vi "shag_start — 5.vi"() -> ()   [LabVIEW 2016]
uses:
  <vilib>/Instr/_visa.llb/VISA Configure Serial Port (Instr).vi
panel:
  out "file":i32
  out "положение в мин 1":i32
  in  "stop":bool
  in  "all":T1(tab)
  out "положение шд":i32(knob) scale=-10.0..190.0
  out "текущее положение":string
  out "положение в минутах 1":string
  in  "Минуты":i32 min=-600 max=11400
  in  "Stop двигатель":bool
  in  "Вращение по градусам +":bool
  in  "Вращение по градусам -":bool
  in  "Вернуться в нулевое положение":bool
  in  "Задать текущее положение нулевым":bool
  in  "Установка минут":bool
  in  "Блокировать зеркало №1":bool
  in  "Выберете COM порт":refnum<visa-resource-name>="COM1"
  in  "Скорость обмена данными":u32(ring)=19200 items=["9600"=9600, "19200"=19200, "38400"=38400, "57600"=57600]
  in  "Число бит на символ":u16=8 min=5 max=8 step=1
  in  "Контроль чётности":enum16{"None", "Odd", "Even", "Mark", "Space"}(ring)
  in  "Стоповый бит":u16(ring)=10 items=["1.0"=10, "1.5"=15, "2.0"=20]
  in  "Контроль переполнения":u16(ring) items=["None"=0, "XON/XOFF"=1, "RTS/CTS"=2, "DTR/DSR"=4]
  # "1 - адресс 1 двигателя\n2 - адресс 2 двигателя\n$0MV\\01+   - запуск всех двигателей в положительном направлении \n$0MS\\00   - остановка всех двигателей\n$0MJ\\04+\\00\\00\\01   - 1 шаг всех двигателей\n$0SS\\01\\10   - скорость 10 для всех двигателей"
  # "Зеркало №1:"
  # "Положение:"
  # "Ренгеновская трубка №2:"
  # "Положение ренгеновской трубк:"
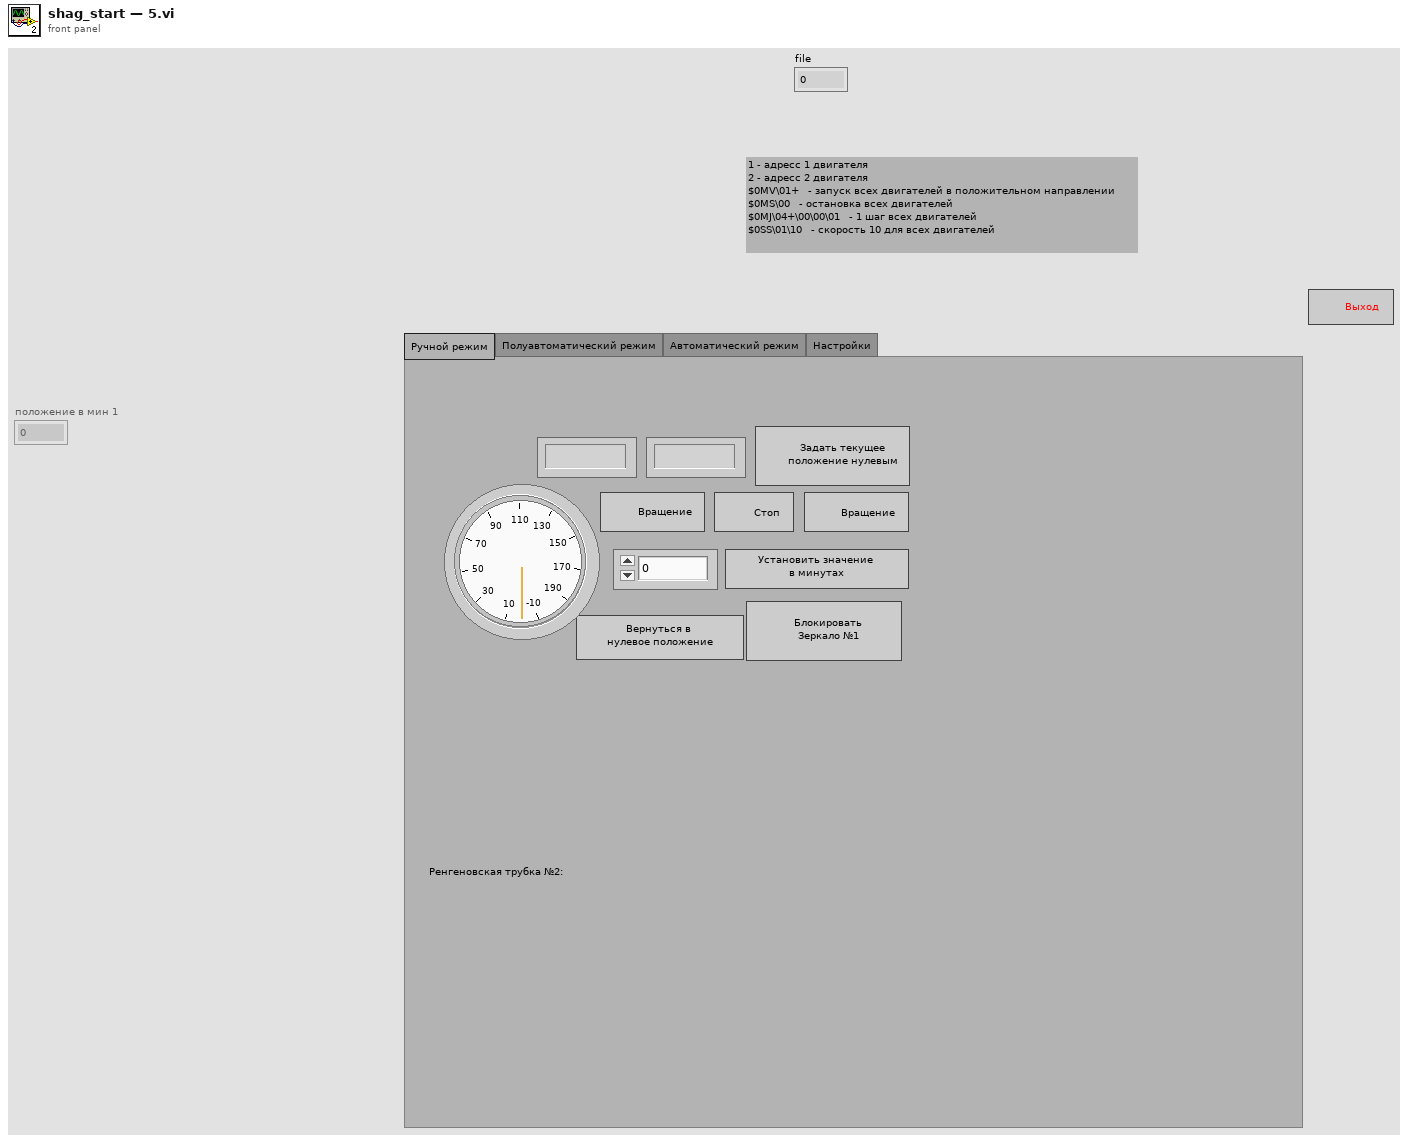
[diagram p1: front panel]
types:
  T1 = enum32{"Ручной режим", "Полуавтоматический режим", "Автоматический режим", "Настройки"}
  T2 = enum16{"open", "replace", "create", "open or create", "replace or create", "replace or create with confirmation"}
  T3 = enum8{"Enabled", "Disabled", "Disabled and Grayed Out"}
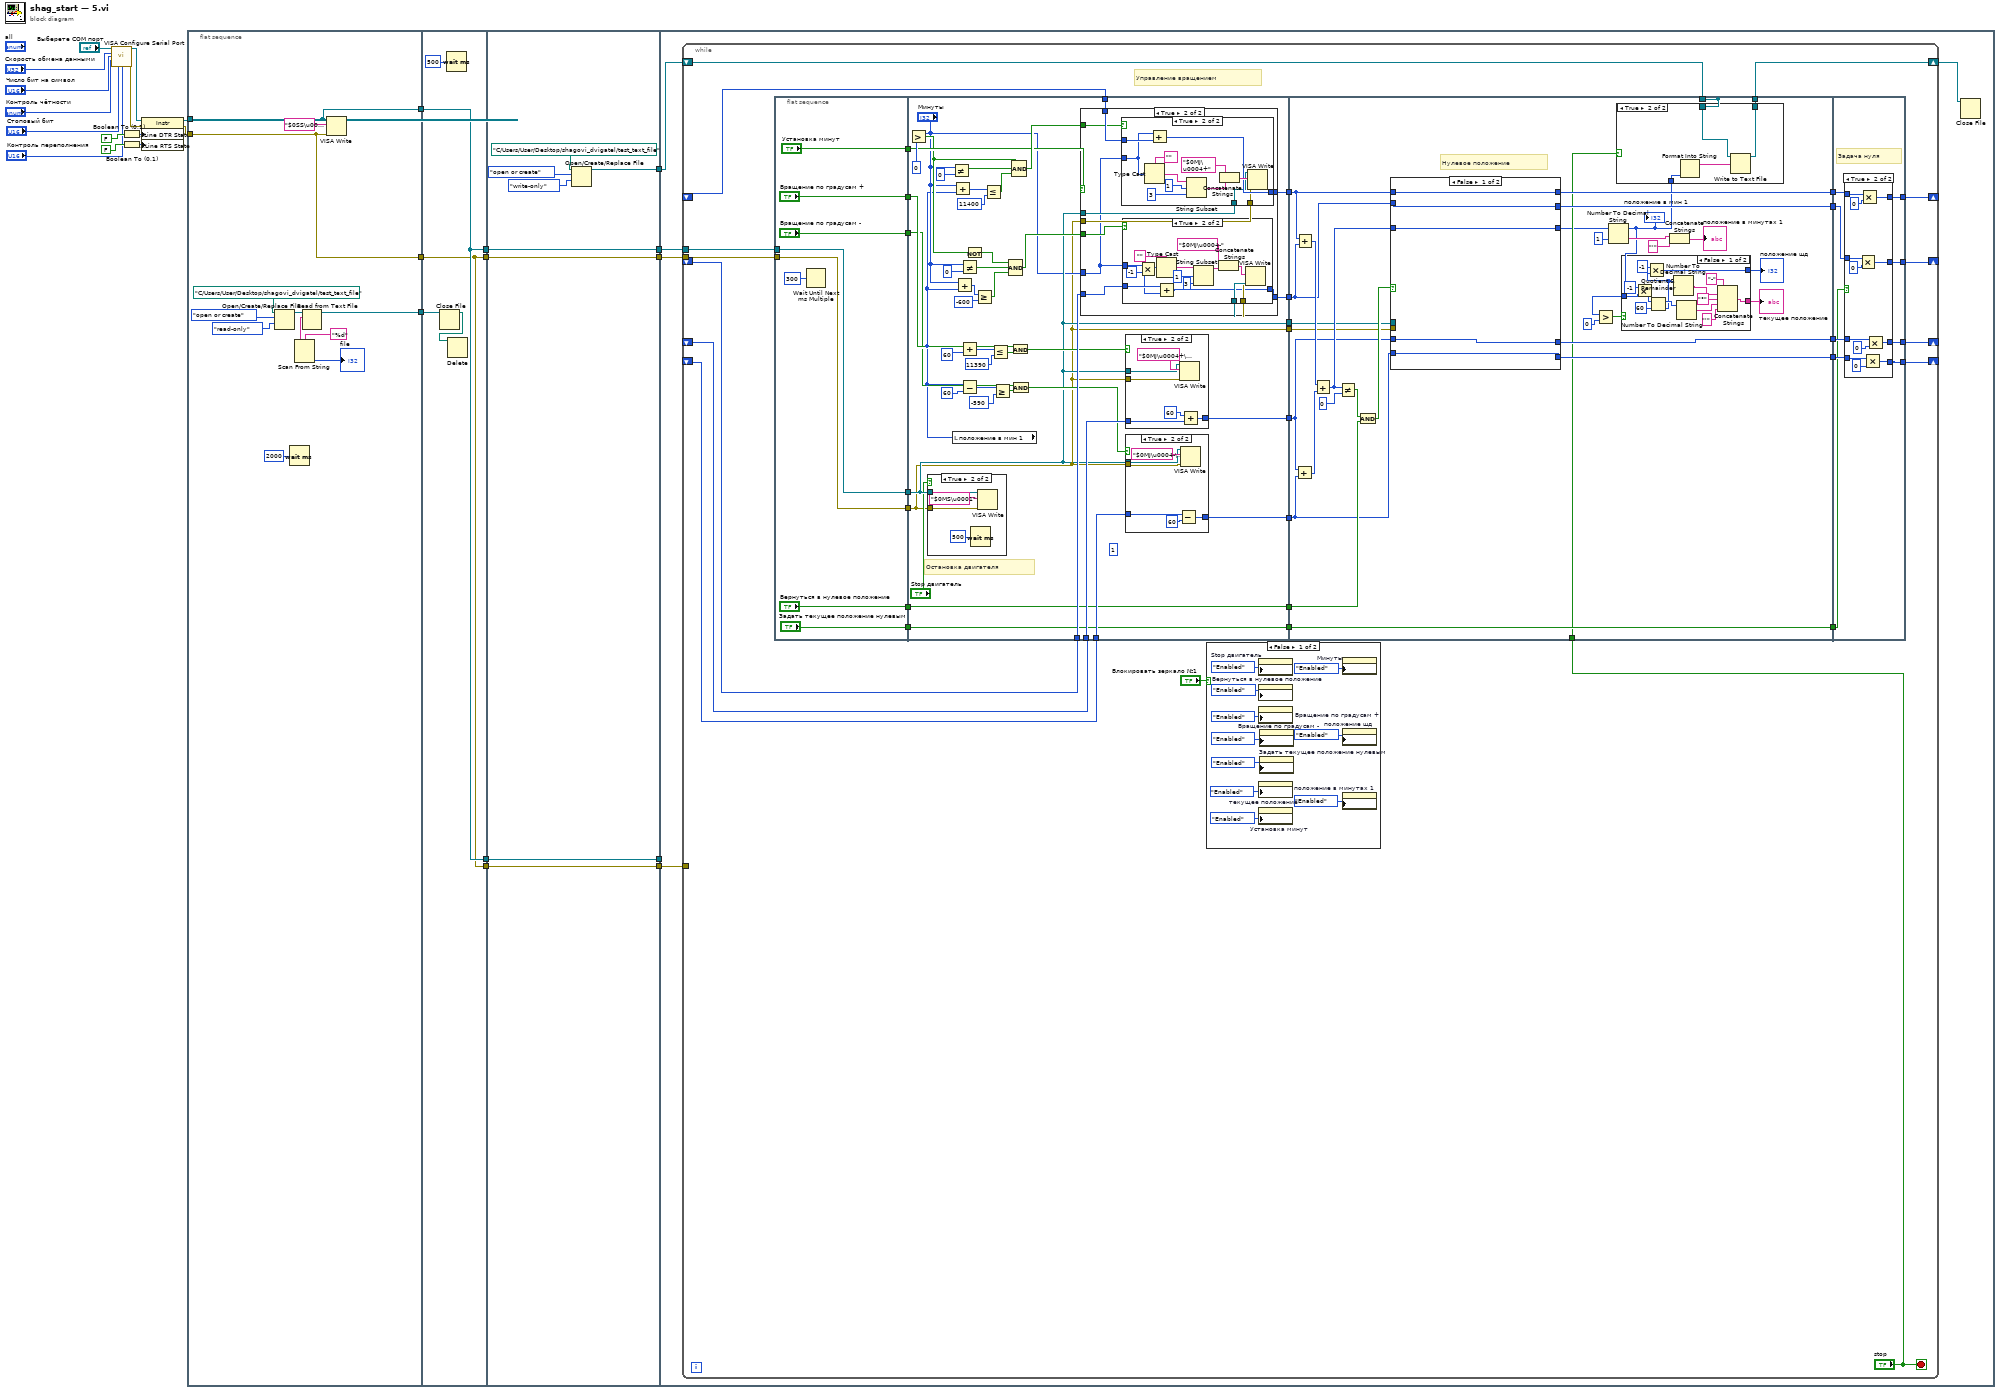
[diagram p0: block diagram]
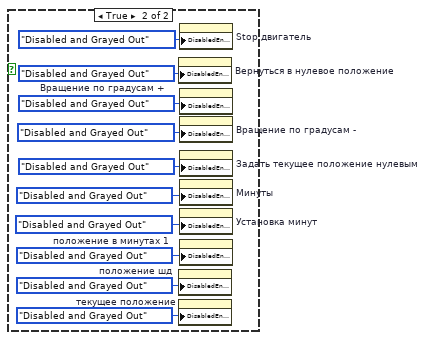
[diagram p2: hidden frame]
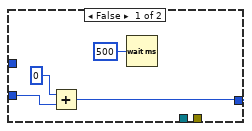
[diagram p4: hidden frame]
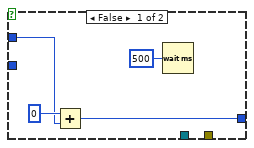
[diagram p5: hidden frame]
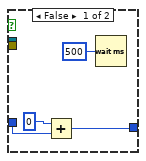
[diagram p7: hidden frame]
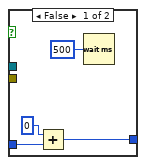
[diagram p8: hidden frame]
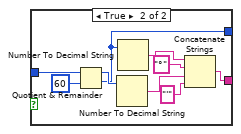
[diagram p10: hidden frame]
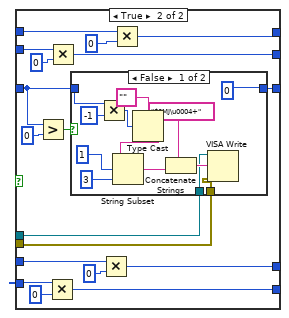
[diagram p11: hidden frame]
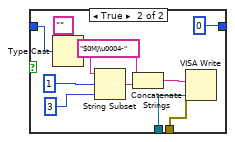
[diagram p12: hidden frame]
diagram:
  n1 = call-poly "VISA Configure Serial Port"("VISA resource name"="Выберете COM порт", "baud rate (9600)"="Скорость обмена данными", "data bits (8)"="Число бит на символ", "parity (0:none)"="Контроль чётности", "stop bits (10: 1 bit)"="Стоповый бит", "flow control (0:none)"="Контроль переполнения") -> ("VISA resource name out"=w24:refnum<visa-resource-name>, "error out"=w23:errorcluster)  [unwired: 8 in]
  n2 = Boolean To (0,1)(Boolean=FALSE ("DTR Write")) -> (0, 1=w25:i16)
  n3 = Boolean To (0,1)(Boolean=FALSE ("DTR Write")) -> (0, 1=w26:i16)
  n4 = property class="Instr"(reference=w24, error in=w23, "Serial Settings:Modem Line Settings:Line DTR State"=w25, "Serial Settings:Modem Line Settings:Line RTS State"=w26) -> (reference out=w22:refnum<visa-resource-name>, error out=w21:errorcluster)
  n5 = flat-sequence {
    tunnel: w22 -> [w37]
    tunnel: w21 -> [w36]
    tunnel: [w37] -> w20
    tunnel: [w36] -> w19
    tunnel: [w30] -> w10
    tunnel: [w42] -> w9
    tunnel: w20 -> [w42]
    tunnel: w19 -> [w41]
    tunnel: [w41] -> w7
    tunnel: [w42] -> w5
    tunnel: [w41] -> w3
    tunnel: w10 -> [w40]
    tunnel: w9 -> [w51]
    tunnel: [w51] -> w8
    tunnel: w7 -> [w50]
    tunnel: [w50] -> w6
    tunnel: w5 -> [w49]
    tunnel: [w49] -> w4
    tunnel: w3 -> [w48]
    tunnel: [w48] -> w2
    tunnel: [w44] -> w1
    tunnel: w8 -> [w56]
    tunnel: w6 -> [w55]
    tunnel: w4 -> [_]
    tunnel: w2 -> [w54]
    tunnel: w1 -> [w53]
    frame #0 {
      n6 = Open/Create/Replace File(file path (use dialog)=path "C:/Users/User/Desktop/shagovi_dvigatel/test_text_file", operation (0:open)=T2."open or create", access (0:read/write)=enum16{"read/write", "read-only", "write-only"}."read-only") -> (refnum out=w29:refnum<file>)  [unwired: 3 in, 2 out]
      n7 = Wait (ms)(milliseconds to wait=u32 2000) -> ()  [unwired: 1 out]
      n8 = Read from Text File(file (use dialog)=w29) -> (refnum out=w30:refnum<file>, text=w33:string)  [unwired: 3 in, 2 out]
      n9 = Scan From String(format string="%d", input string=w33) -> (output 1=→"file":i32)  [unwired: 3 in, 3 out]
      n10 = VISA Write(VISA resource name=w37, write buffer="$0SS\u0001\u0010", error in (no error)=w36) -> ()  [unwired: 3 out]
    }
    frame #1 {
      n11 = Close File(refnum=w40) -> (path=w39:path)  [unwired: 1 in, 1 out]
      n12 = Wait (ms)(milliseconds to wait=u32 500) -> ()  [unwired: 1 out]
      n13 = Delete(path (use dialog)=w39) -> ()  [unwired: 4 in, 3 out]
    }
    frame #2 {
      n14 = Open/Create/Replace File(file path (use dialog)=path "C:/Users/User/Desktop/shagovi_dvigatel/test_text_file", operation (0:open)=T2."open or create", access (0:read/write)=enum16{"read/write", "read-only", "write-only"}."write-only") -> (refnum out=w44:refnum<file>)  [unwired: 3 in, 2 out]
    }
    frame #3 {
      n15 = while {
        tunnel: w56 -> [w66]
        tunnel: w55 -> [w65]
        shift-right: [w61] -> _
        shift-left: _ -> [w70]
        shift-right: [w62] -> _
        shift-left: _ -> [w69]
        shift-right: [w63] -> _
        shift-left: _ -> [w68]
        shift-right: [w64] -> _
        shift-left: _ -> [w67]
        tunnel: w54 -> [_]
        shift-right: [w57] -> w52
        shift-left: w53 -> [w58]
        stop <- "stop" stop-if-true
        # "Управление вращением"
        n16 = flat-sequence {
          tunnel: w65 -> [w117]
          tunnel: w66 -> [w118]
          tunnel: [w118] -> w90
          tunnel: [w117] -> w89
          tunnel: ["Вращение по градусам +"] -> w88
          tunnel: ["Вращение по градусам -"] -> w87
          tunnel: ["Вернуться в нулевое положение"] -> w86
          tunnel: ["Задать текущее положение нулевым"] -> w85
          tunnel: ["Установка минут"] -> w84
          tunnel: w90 -> [w138]
          tunnel: w89 -> [w120]
          tunnel: [w161] -> w83
          tunnel: w70 -> [w158]
          tunnel: w69 -> [w160]
          tunnel: [w159] -> w82
          tunnel: w68 -> [w157]
          tunnel: w67 -> [w156]
          tunnel: w88 -> [w142]
          tunnel: w87 -> [w141]
          tunnel: [w155] -> w81
          tunnel: [w154] -> w80
          tunnel: [w139] -> w79
          tunnel: w86 -> [w139]
          tunnel: [w120] -> w78
          tunnel: [w138] -> w77
          tunnel: [w137] -> w76
          tunnel: w85 -> [w137]
          tunnel: w84 -> [w131]
          tunnel: w83 -> [w239]
          tunnel: w82 -> [w240]
          tunnel: [w260] -> w75
          tunnel: [w258] -> w74
          tunnel: w81 -> [w241]
          tunnel: w80 -> [w242]
          tunnel: [w248] -> w73
          tunnel: [w256] -> w72
          tunnel: w79 -> [w252]
          tunnel: w78 -> [w247]
          tunnel: w77 -> [w246]
          tunnel: w76 -> [w244]
          tunnel: [w244] -> w71
          tunnel: [w233] -> _
          tunnel: "stop" -> [w236]
          tunnel: w58 -> [w233]
          tunnel: [w232] -> w57
          tunnel: [w344] -> w61
          tunnel: [w341] -> w62
          tunnel: w75 -> [w343]
          tunnel: w74 -> [w342]
          tunnel: [w340] -> w63
          tunnel: [w339] -> w64
          tunnel: w73 -> [w338]
          tunnel: w72 -> [w337]
          tunnel: w71 -> [w336]
          frame #0 {
            n17 = Wait Until Next ms Multiple(millisecond multiple=u32 300) -> ()  [unwired: 1 out]
          }
          frame #1 {
            (unwired) 1
            # "Остановка двигателя"
            n18 = Greater?(x="Минуты", y=0) -> (0:w129:bool)
            n19 = case shown="True" "Stop двигатель" {
              tunnel: w138 -> [_ w208]
              tunnel: w120 -> [_ w207]
              frame False {
              }
              frame True {
                n20 = Wait (ms)(milliseconds to wait=u32 500) -> ()  [unwired: 1 out]
                n21 = VISA Write(VISA resource name=w208, write buffer="$0MS\u0001", error in (no error)=w207) -> ()  [unwired: 3 out]
              }
            }
            n22 = Not Equal?(x="Минуты", y=0) -> (x != y?=w128:bool)
            n23 = local read "положение в мин 1"() -> (w119:i32)
            n24 = Add(x="Минуты", y=w119) -> (x+y=w152:i32)
            n25 = Add(x="Минуты", y=w119) -> (x+y=w123:i32)
            n26 = Not Equal?(x="Минуты", y=0) -> (x != y?=w126:bool)
            n27 = Add(x=w119, y=60) -> (x+y=w147:i32)
            n28 = Subtract(x=w119, y=60) -> (x-y=w134:i32)
            n29 = Not(x=w129) -> (.not. x?=w130:bool)
            n30 = Greater Or Equal?(x=w123, y=-600) -> (x >= y?=w124:bool)
            n31 = Less Or Equal?(x=w152, y=11400) -> (x <= y?=w127:bool)
            n32 = Less Or Equal?(x=w147, y=11390) -> (x <= y?=w144:bool)
            n33 = Greater Or Equal?(x=w134, y=-590) -> (x >= y?=w135:bool)
            n34 = Compound Arithmetic op=AND(w130, w126, w124) -> (w148:bool)
            n35 = And(x=w142, y=w144) -> (x .and. y?=w143:bool)
            n36 = And(x=w141, y=w135) -> (x .and. y?=w140:bool)
            n37 = Compound Arithmetic op=AND(w129, w128, w127) -> (w150:bool)
            n38 = case shown="True" w131 {
              tunnel: [w163 w172] -> w161
              tunnel: w160 -> [w162 w171]
              tunnel: [w162 w170] -> w159
              tunnel: w158 -> [w163 w169]
              tunnel: w150 -> [_ w168]
              tunnel: w148 -> [_ w167]
              tunnel: w120 -> [_ w166]
              tunnel: w138 -> [_ w165]
              tunnel: "Минуты" -> [_ w164]
              frame False {
              }
              frame True {
                n39 = case shown="True" w168 {
                  tunnel: [w193 w199] -> w172
                  tunnel: w169 -> [w192 w198]
                  tunnel: w166 -> [_ w197]
                  tunnel: w165 -> [_ w196]
                  tunnel: w164 -> [_ w195]
                  frame False {
                    n40 = Add(x=0, y=w192) -> (x+y=w193:i32)
                    n41 = Wait (ms)(milliseconds to wait=u32 500) -> ()  [unwired: 1 out]
                  }
                  frame True {
                    n42 = Type Cast(type="", x=w195) -> (*(type *) &x=w202:string)
                    n43 = Add(x=w195, y=w198) -> (x+y=w199:i32)
                    n44 = String Subset(string=w202, offset (0)=1, length (rest)=3 ("length (rest)")) -> (substring=w201:string)
                    n45 = Concatenate Strings("$0MJ\u0004+" ("write buffer"), w201) -> (w205:string)
                    n46 = VISA Write(VISA resource name=w196, write buffer=w205, error in (no error)=w197) -> ()  [unwired: 3 out]
                  }
                }
                n47 = case shown="True" w167 {
                  tunnel: [w175 w181] -> w170
                  tunnel: w171 -> [w174 w180]
                  tunnel: w165 -> [_ w183]
                  tunnel: w166 -> [_ w182]
                  tunnel: w164 -> [_ w177]
                  frame False {
                    n48 = Add(x=0, y=w174) -> (x+y=w175:i32)
                    n49 = Wait (ms)(milliseconds to wait=u32 500) -> ()  [unwired: 1 out]
                  }
                  frame True {
                    n50 = Multiply(x=w177, y=-1) -> (x*y=w179:i32)
                    n51 = Type Cast(type="", x=w179) -> (*(type *) &x=w186:string)
                    n52 = Add(x=w180, y=w177) -> (x+y=w181:i32)
                    n53 = String Subset(string=w186, offset (0)=1, length (rest)=3 ("length (rest)")) -> (substring=w185:string)
                    n54 = Concatenate Strings("$0MJ\u0004-" ("write buffer"), w185) -> (w189:string)
                    n55 = VISA Write(VISA resource name=w183, write buffer=w189, error in (no error)=w182) -> ()  [unwired: 3 out]
                  }
                }
              }
            }
            n56 = case shown="True" w143 {
              tunnel: [w223 w230] -> w155
              tunnel: w157 -> [w222 w225]
              tunnel: w138 -> [_ w226]
              tunnel: w120 -> [_ w227]
              frame False {
                n57 = Add(x=0, y=w222) -> (x+y=w223:i32)
                n58 = Wait (ms)(milliseconds to wait=u32 500) -> ()  [unwired: 1 out]
              }
              frame True {
                n59 = VISA Write(VISA resource name=w226, write buffer="$0MJ\u0004+\u0000\u0000<", error in (no error)=w227) -> ()  [unwired: 3 out]
                n60 = Add(x=60, y=w225) -> (x+y=w230:i32)
              }
            }
            n61 = case shown="True" w140 {
              tunnel: [w213 w216] -> w154
              tunnel: w156 -> [w212 w215]
              tunnel: w138 -> [_ w219]
              tunnel: w120 -> [_ w218]
              frame False {
                n62 = Add(x=0, y=w212) -> (x+y=w213:i32)
                n63 = Wait (ms)(milliseconds to wait=u32 500) -> ()  [unwired: 1 out]
              }
              frame True {
                n64 = Subtract(x=w215, y=60 ("x")) -> (x-y=w216:i32)
                n65 = VISA Write(VISA resource name=w219, write buffer="$0MJ\u0004-\u0000\u0000<", error in (no error)=w218) -> ()  [unwired: 3 out]
              }
            }
          }
          frame #2 {
            # "Нулевое положение"
            n66 = Add(x=w241, y=w242) -> (x+y=w253:i32)
            n67 = Add(x=w239, y=w240) -> (x+y=w257:i32)
            n68 = Add(x=w257, y=w253) -> (x+y=w250:i32)
            n69 = Not Equal?(x=w250, y=0 ("x")) -> (x != y?=w249:bool)
            n70 = And(x=w249, y=w252) -> (x .and. y?=w259:bool)
            n71 = case shown="False" w259 {
              tunnel: [w289 w311] -> w231
              tunnel: w239 -> [w293 w308]
              tunnel: [w293 w307] -> w260
              tunnel: [w292 w306] -> w258
              tunnel: w250 -> [w289 w300]
              tunnel: [w290 w302] -> w256
              tunnel: [w291 w299] -> w248
              tunnel: w240 -> [w292 w298]
              tunnel: w247 -> [_ w297]
              tunnel: w246 -> [_ w296]
              tunnel: w241 -> [w291 w295]
              tunnel: w242 -> [w290 w294]
              frame False {
              }
              frame True {
                n72 = Greater?(x=w300, y=0) -> (0:w301:bool)
                n73 = Multiply(x=w294, y=0) -> (x*y=w302:i32)
                n74 = Multiply(x=w298, y=0) -> (x*y=w306:i32)
                n75 = case shown="False" w301 {
                  tunnel: w300 -> [w316 w329]
                  tunnel: [0 0] -> w311
                  tunnel: w296 -> [w313 w326]
                  tunnel: w297 -> [w312 w325]
                  frame False {
                    n76 = Multiply(x=w316, y=-1) -> (x*y=w314:i32)
                    n77 = Type Cast(type="", x=w314) -> (*(type *) &x=w320:string)
                    n78 = String Subset(string=w320, offset (0)=1, length (rest)=3 ("length (rest)")) -> (substring=w319:string)
                    n79 = Concatenate Strings("$0MJ\u0004+" ("write buffer"), w319) -> (w323:string)
                    n80 = VISA Write(VISA resource name=w313, write buffer=w323, error in (no error)=w312) -> ()  [unwired: 3 out]
                  }
                  frame True {
                    n81 = Type Cast(type="", x=w329) -> (*(type *) &x=w332:string)
                    n82 = String Subset(string=w332, offset (0)=1, length (rest)=3 ("length (rest)")) -> (substring=w331:string)
                    n83 = Concatenate Strings("$0MJ\u0004-" ("write buffer"), w331) -> (w327:string)
                    n84 = VISA Write(VISA resource name=w326, write buffer=w327, error in (no error)=w325) -> ()  [unwired: 3 out]
                  }
                }
                n85 = Multiply(x=w295, y=0) -> (x*y=w299:i32)
                n86 = Multiply(x=w308, y=0) -> (x*y=w307:i32)
              }
            }
            "положение в мин 1" <- w231
            n87 = Greater?(x=w231, y=0) -> (0:w255:bool)
            n88 = Number To Decimal String(number=w231, width (-)=i16 1) -> (decimal integer string=w235:string)
            n89 = case shown="True" w236 {
              tunnel: w233 -> [w261 w263]
              tunnel: w231 -> [_ w264]
              tunnel: [w261 w262] -> w232
              frame False {
              }
              frame True {
                n90 = Format Into String(w264) -> (resulting string=w265:string)  [unwired: 3 in, 1 out]
                n91 = Write to Text File(file (use dialog)=w263, text=w265) -> (refnum out=w262:refnum<file>)  [unwired: 2 in, 2 out]
              }
            }
            n92 = case shown="False" w255 {
              tunnel: w231 -> [w272 w288]
              tunnel: [w276 w282] -> w245
              tunnel: [w266 w280] -> w243
              frame False {
                n93 = Multiply(x=-1, y=w272) -> (x*y=w271:i32)
                n94 = Quotient & Remainder(x=w271, y=60) -> (x-y*floor(x/y)=w275:i32, floor(x/y)=w267:i32)
                n95 = Multiply(x=-1, y=w267) -> (x*y=w266:i32)
                n96 = Number To Decimal String(number=w267) -> (decimal integer string=w273:string)  [unwired: 1 in]
                n97 = Number To Decimal String(number=w275) -> (decimal integer string=w274:string)  [unwired: 1 in]
                n98 = Concatenate Strings("-" ("string"), w273, "°" ("string"), w274, "'" ("string")) -> (w276:string)
              }
              frame True {
                n99 = Quotient & Remainder(x=w288, y=60) -> (x-y*floor(x/y)=w281:i32, floor(x/y)=w280:i32)
                n100 = Number To Decimal String(number=w281) -> (decimal integer string=w283:string)  [unwired: 1 in]
                n101 = Number To Decimal String(number=w280) -> (decimal integer string=w284:string)  [unwired: 1 in]
                n102 = Concatenate Strings(w284, "°" ("string"), w283, "'" ("string")) -> (w282:string)
              }
            }
            "положение шд" <- w243
            "текущее положение" <- w245
            n103 = Concatenate Strings(w235, "'" ("string")) -> (→"положение в минутах 1":string)
          }
          frame #3 {
            # "Задача нуля"
            n104 = case shown="True" w336 {
              tunnel: [w348 w359] -> w344
              tunnel: w343 -> [w348 w360]
              tunnel: w342 -> [w347 w356]
              tunnel: [w347 w355] -> w341
              tunnel: [w346 w352] -> w340
              tunnel: [w345 w351] -> w339
              tunnel: w338 -> [w346 w350]
              tunnel: w337 -> [w345 w349]
              frame False {
              }
              frame True {
                n105 = Multiply(x=w356, y=0) -> (x*y=w355:i32)
                n106 = Multiply(x=w360, y=0) -> (x*y=w359:i32)
                n107 = Multiply(x=w349, y=0) -> (x*y=w351:i32)
                n108 = Multiply(x=w350, y=0) -> (x*y=w352:i32)
              }
            }
          }
        }
        n109 = case shown="False" "Блокировать зеркало №1" {
          frame False {
            n110 = property on="Stop двигатель" class="Bool"("DisabledEnum"=T3."Enabled" ("Disabled")) -> ()  [unwired: 2 in, 2 out]
            n111 = property on="Вернуться в нулевое положение" class="Bool"("DisabledEnum"=T3."Enabled" ("Disabled")) -> ()  [unwired: 2 in, 2 out]
            n112 = property on="Вращение по градусам +" class="Bool"("DisabledEnum"=T3."Enabled" ("Disabled")) -> ()  [unwired: 2 in, 2 out]
            n113 = property on="текущее положение" class="Str"("DisabledEnum"=T3."Enabled" ("Disabled")) -> ()  [unwired: 2 in, 2 out]
            n114 = property on="Установка минут" class="Bool"("DisabledEnum"=T3."Enabled" ("Disabled")) -> ()  [unwired: 2 in, 2 out]
            n115 = property on="Вращение по градусам -" class="Bool"("DisabledEnum"=T3."Enabled" ("Disabled")) -> ()  [unwired: 2 in, 2 out]
            n116 = property on="Задать текущее положение нулевым" class="Bool"("DisabledEnum"=T3."Enabled" ("Disabled")) -> ()  [unwired: 2 in, 2 out]
            n117 = property on="Минуты" class="DigNum (strict)"("DisabledEnum"=T3."Enabled" ("Disabled")) -> ()  [unwired: 2 in, 2 out]
            n118 = property on="положение шд" class="Knob (strict)"("DisabledEnum"=T3."Enabled" ("Disabled")) -> ()  [unwired: 2 in, 2 out]
            n119 = property on="положение в минутах 1" class="Str"("DisabledEnum"=T3."Enabled" ("Disabled")) -> ()  [unwired: 2 in, 2 out]
          }
          frame True {
            n120 = property on="Вернуться в нулевое положение" class="Bool"("DisabledEnum"=T3."Disabled and Grayed Out" ("Disabled")) -> ()  [unwired: 2 in, 2 out]
            n121 = property on="положение шд" class="Knob (strict)"("DisabledEnum"=T3."Disabled and Grayed Out" ("Disabled")) -> ()  [unwired: 2 in, 2 out]
            n122 = property on="текущее положение" class="Str"("DisabledEnum"=T3."Disabled and Grayed Out" ("Disabled")) -> ()  [unwired: 2 in, 2 out]
            n123 = property on="Stop двигатель" class="Bool"("DisabledEnum"=T3."Disabled and Grayed Out" ("Disabled")) -> ()  [unwired: 2 in, 2 out]
            n124 = property on="Вращение по градусам +" class="Bool"("DisabledEnum"=T3."Disabled and Grayed Out" ("Disabled")) -> ()  [unwired: 2 in, 2 out]
            n125 = property on="Вращение по градусам -" class="Bool"("DisabledEnum"=T3."Disabled and Grayed Out" ("Disabled")) -> ()  [unwired: 2 in, 2 out]
            n126 = property on="Задать текущее положение нулевым" class="Bool"("DisabledEnum"=T3."Disabled and Grayed Out" ("Disabled")) -> ()  [unwired: 2 in, 2 out]
            n127 = property on="Минуты" class="DigNum (strict)"("DisabledEnum"=T3."Disabled and Grayed Out" ("Disabled")) -> ()  [unwired: 2 in, 2 out]
            n128 = property on="Установка минут" class="Bool"("DisabledEnum"=T3."Disabled and Grayed Out" ("Disabled")) -> ()  [unwired: 2 in, 2 out]
            n129 = property on="положение в минутах 1" class="Str"("DisabledEnum"=T3."Disabled and Grayed Out" ("Disabled")) -> ()  [unwired: 2 in, 2 out]
          }
        }
      }
      n130 = Close File(refnum=w52) -> ()  [unwired: 1 in, 2 out]
    }
  }
